vi "TagBrowse.vi"(7 "LabVIEW Web Service Request":refnum<class "Web Request.lvclass">) -> ()   [LabVIEW 2013]
doc: "TagBrowse returns a list of the name, type, and permissions of every tag in the CVT."
uses:
  <vilib>/wsapi/Web Request.lvclass
  <vilib>/NI/Tag Bus Module Framework/channel/TBM channel.lvclass
  <vilib>/NI/TagWebClient/API/JSON Formats/TagBrowse Results.ctl
  <vilib>/NI/TagWebClient/API/Logical Groups/Tags in Group.ctl
  <vilib>/NI/TagWebClient/API/Logical Groups/tags.ctl
  <vilib>/NI/Tag Bus/tag/tag descriptor.lvclass/tag descriptor.ctl
  <vilib>/NI/Tag Bus Module Framework/channel/TBM channel.lvclass/TBM channel.ctl
  <vilib>/NI/Tag Bus/tag/read tag name.vi
  <vilib>/NI/Tag Bus Module Framework/channel/Read channel classification.vi
  <vilib>/NI/Tag Bus/tag/count types.vi
  <vilib>/NI/Tag Bus/tag/index to type.vi
  <vilib>/NI/TagWebClient/API/tagweb client API.lvlib
  <vilib>/NI/Tag Bus/tag/tag descriptor.lvclass
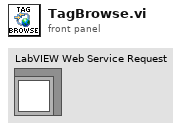
[diagram p1: front panel]
types:
  T1 = typedef "tagweb client API.lvlib/TagBrowse Results.ctl" = cluster{"groupName":string, "Tags":T2[]}
  T2 = typedef "tagweb client API.lvlib/Tags in Group.ctl" = cluster{"type":string, "tags":T3[]}
  T3 = typedef "tagweb client API.lvlib/tags.ctl" = cluster{"tagName":string, "permissions":string}
  T4 = typedef "tag bus.lvlib/tag descriptor.lvclass/Data Type.ctl" = enum16{"Double", "Single", "I64", "I32", "I16", "I8", "U64", "U32", "U16", "U8", "Boolean", "String", "Array of Double", "Array of Single", "Array of I64", "Array of I32", "Array of I16", "Array of I8", "Array of U64", "Array of U32", "Array of U16", "Array of U8", "Array of Boolean", "Array of String"}
  T5 = typedef "TBM channel.lvclass/channel classification.ctl" = enum16{"input data", "output data", "processing parameter", "processing result"}
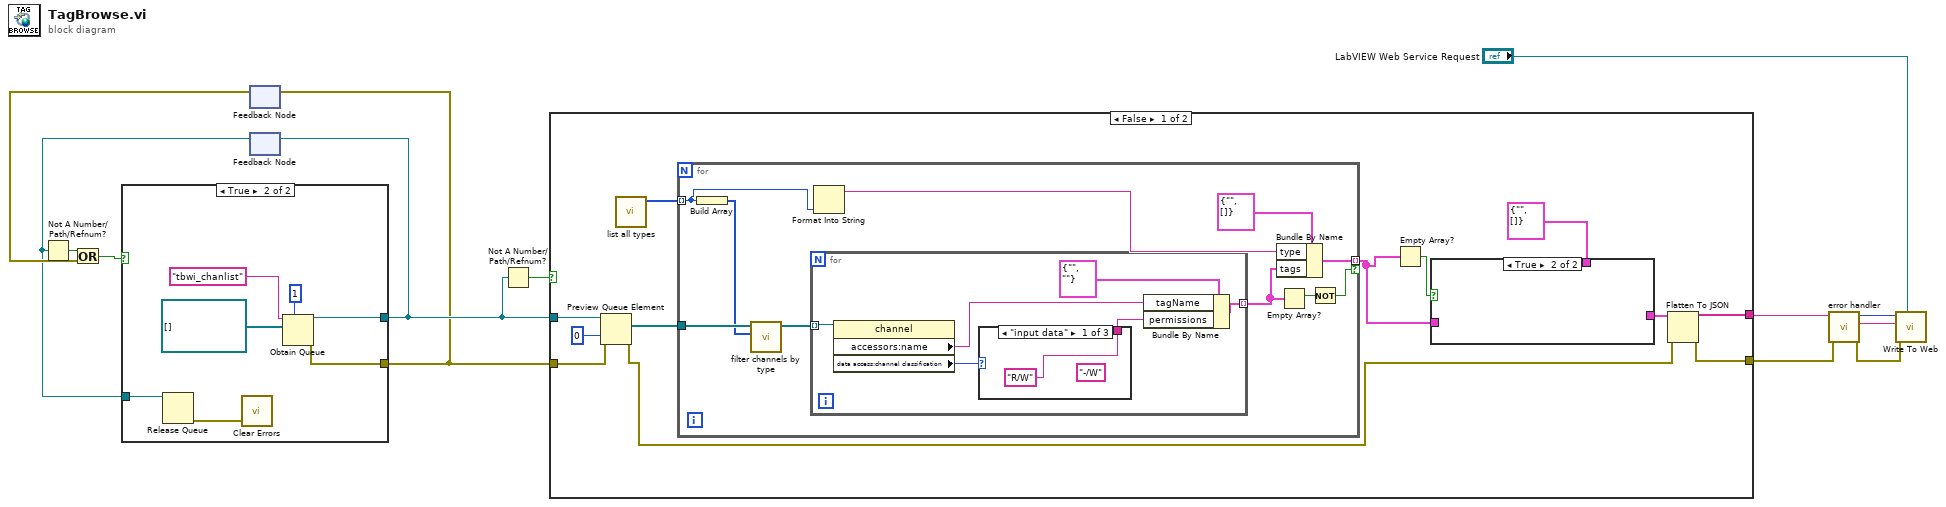
[diagram p0: block diagram]
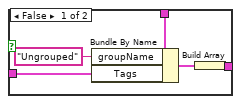
[diagram p3: hidden frame]
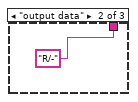
[diagram p4: hidden frame]
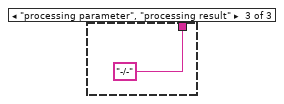
[diagram p5: hidden frame]
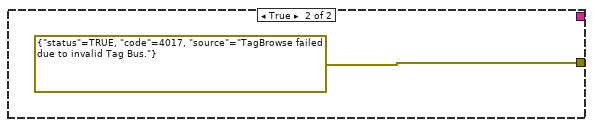
[diagram p6: hidden frame]
diagram:
  n1 = feedback #1() -> (w3:errorcluster)  [unwired: 1 in]
  n2 = feedback #2() -> (w1:refnum<queue>)  [unwired: 1 in]
  n3 = Not A Number/Path/Refnum?(number/path/refnum=w1) -> (NaN/Path/Refnum?=w4:bool)
  n4 = Or(x=w4, y=w3) -> (x .or. y?=w2:bool)
  n5 = case shown="True" w2 {
    tunnel: [_ w18] -> w5
    tunnel: [w14 w17] -> w6
    tunnel: w1 -> [w14 w15]
    frame False {
    }
    frame True {
      n6 = Release Queue(queue=w15) -> (error out=w16:errorcluster)  [unwired: 2 in, 2 out]
      n7 = call <vilib>:"Clear Errors.vi"("error in (no error)"=w16) -> ()  [unwired: 6 in, 1 out]
      n8 = Obtain Queue(max queue size (-1, unlimited)=1, name (unnamed)="tbwi_chanlist", element data type=refnum<class "TBM channel.lvclass">[] [] ("channels in")) -> (queue out=w17:refnum<queue>, error out=w18:errorcluster)  [unwired: 2 in, 1 out]
    }
  }
  n9 = feedback-in #1(w5) -> ()
  n10 = feedback-in #2(w6) -> ()
  n11 = Not A Number/Path/Refnum?(number/path/refnum=w6) -> (NaN/Path/Refnum?=w8:bool)
  n12 = case shown="False" w8 {
    tunnel: w5 -> [w33 _]
    tunnel: w6 -> [w32 _]
    tunnel: [w28 errorcluster {"status"=TRUE, "code"=4017, "source"="TagBrowse failed due to invalid Tag Bus."} ("error out")] -> w13
    tunnel: [w29 _] -> w12
    frame False {
      n13 = Preview Queue Element(queue=w32, timeout in ms (-1)=0, error in (no error)=w33) -> (element=w25:refnum<class "TBM channel.lvclass">[], error out=w27:errorcluster)  [unwired: 2 out]
      n14 = call <vilib>:"list all types.vi"() -> ("all types"=w26:T4[])  [unwired: 11 in]
      n15 = for {
        tunnel: w26 -> [w48] mode=indexing
        tunnel: w25 -> [w45]
        tunnel: [w46] -> w23 mode=indexing if=w40
        n16 = Build Array(w48) -> (w43:T4[])
        n17 = call <vilib>:"filter channels by type.vi"("allowed types"=w43, "channels in"=w45) -> ("channels out"=w44:refnum<class "TBM channel.lvclass">[])  [unwired: 9 in]
        n18 = for {
          tunnel: [w54] -> w42 mode=indexing
          tunnel: w44 -> [w53] mode=indexing
          n19 = property class="channel"(reference=w53) -> ("accessors:name"=w52:string, "data access:channel classification"=w51:T5)  [unwired: 1 in, 2 out]
          n20 = case shown="\"input data\"" w51 {
            tunnel: ["R/W" "R/-" "-/-"] -> w50
            frame "input data" {
              (unwired) "-/W"
            }
            frame "output data" {
            }
            frame "processing parameter", "processing result" {
            }
          }
          n21 = Bundle By Name(cluster=T3 {"tagName"="", "permissions"=""} ("tags"), "tagName"=w52, "permissions"=w50) -> (w54:T3)
        }
        n22 = Format Into String(w48) -> (resulting string=w47:string)  [unwired: 3 in, 1 out]
        n23 = Bundle By Name(cluster=T2 {"type"="", "tags"=[]} ("Cluster"), "type"=w47, "tags"=w42) -> (w46:T2)
        n24 = Empty Array?(array=w42) -> (empty?=w41:bool)
        n25 = Not(x=w41) -> (.not. x?=w40:bool)
      }
      n26 = Empty Array?(array=w23) -> (empty?=w22:bool)
      n27 = case shown="True" w22 {
        tunnel: [w36 _] -> w30
        tunnel: T1 {"groupName"="", "Tags"=[]} ("TagBrowse Results") -> [w35 _]
        tunnel: w23 -> [w34 _]
        frame False {
          n28 = Bundle By Name(cluster=w35, "groupName"="Ungrouped", "Tags"=w34) -> (w37:T1)
          n29 = Build Array(w37) -> (w36:T1[])
        }
        frame True {
        }
      }
      n30 = Flatten To JSON(anything=w30, error in (no error)=w27) -> (JSON string=w29:string, 11:w28:errorcluster)  [unwired: 1 in]
    }
    frame True {
    }
  }
  n31 = call "error handler.vi"("error in (no error)"=w13, "Success Message"=w12) -> ("error out"=w11:errorcluster, "Response String"=w9:string, "Response Code"=w10:i32)  [unwired: 7 in]
  n32 = call <vilib>:"Write To Web.vi"("Web Request in"="LabVIEW Web Service Request", "error in"=w11, "Response String"=w9, "Response Code"=w10) -> ()  [unwired: 8 in]
